vi "Sequencer Trigger Manually.vi"(8 "error in (no error)":errorcluster, 10 "Instance (1)":i32=1, 11 "VISA resource name":refnum<visa-resource-name>) -> (0 "error out":errorcluster, 3 "VISA resource name out":refnum<visa-resource-name>)   [LabVIEW 2020, in "Rohde&Schwarz CMXP GPRF.lvlib"]
doc: "Triggers the transition to the next sequencer list entry manually.\n\nAttribute:\nRSCMXPGPRF_ATTR_SEQUENCER_TRIGGER_MANUALLY\n\nRemote-control command:\nTRIGger:GPRF:GEN<i>:SEQuencer:MANual:EXECute"
uses:
  <instrlib>/Rohde&Schwarz CMXP GPRF/Rohde&Schwarz CMXP GPRF.lvlib
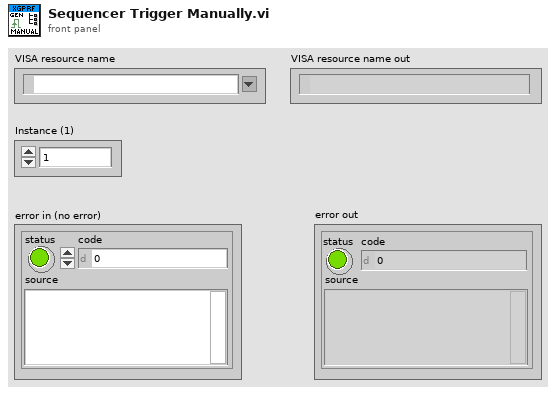
[diagram p1: front panel]
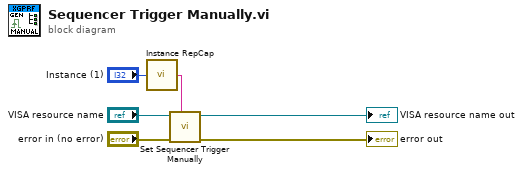
[diagram p0: block diagram]
diagram:
  n1 = call <instrlib>:"Instance RepCap.vi"("Instance in"="Instance (1)") -> ("Instance out"=w1:string)
  n2 = call "Set Sequencer Trigger Manually"("Repeated Capabilities"=w1, "error in (no error)"="error in (no error)", "instrument handle"="VISA resource name") -> ("error out"=→"error out":errorcluster, "instrument handle out"=→"VISA resource name out":refnum<visa-resource-name>)  [unwired: 7 in]
